vi "createCommandParameters.vi"(8 "error in (no error)":errorcluster, 9 "value":variant, 10 "command":T1, 11 "CoolerSerialCommand in":refnum<class "CoolerSerialCommand.lvclass">) -> (0 "error out":errorcluster, 1 "commandName":string, 2 "commandId":string, 3 "CoolerSerialCommand out":refnum<class "CoolerSerialCommand.lvclass">, 5 "cmdData":string)   [LabVIEW 2016, in "CoolerSerialCommand.lvclass"]
uses:
  CoolerSerialCommand.lvclass
  typedefs/CoolerCommands.ctl
  typedefs/dataType.ctl
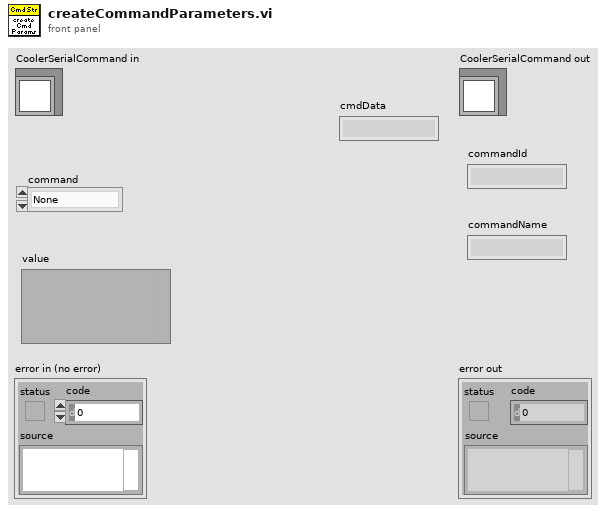
[diagram p1: front panel]
types:
  T1 = typedef "CoolerCommands.ctl" = enum16{"None", "SetExternSensorStatus", "SetChillerStatus", "SetControlSensor", "SetControlTemperature", "SetHighSupplyTempWarning", "SetLowSupplyTemperatureWarning", "SetHighAmbientTemperatureWarning", "SetLowAmbienTemperatureWarning", "SetLowProcessFlowWarning", "SetHighSupplyTemperatureAlarm", "SetLowSupplyTemperatureAlarm", "SetHighAmbientTemperatureAlarm", "SetLowAmbientTemperatureAlarm", "SetLowProcessFlowAlarm"}
  T2 = typedef "dataType.ctl" = enum16{"Temperature", "Flow", "ControlSensor", "ExternalSensorStatus", "ChillerStatus"}
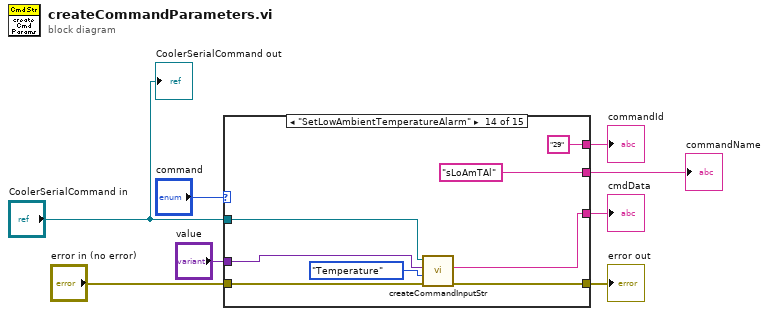
[diagram p0: block diagram]
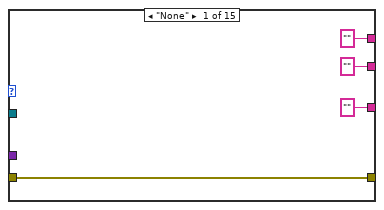
[diagram p2: hidden frame]
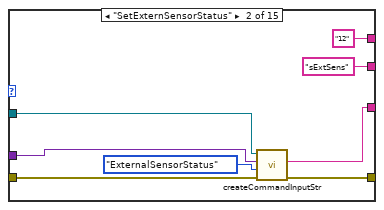
[diagram p3: hidden frame]
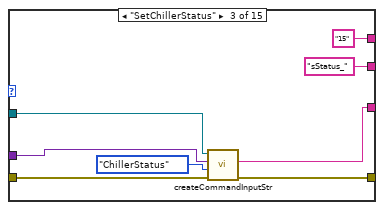
[diagram p4: hidden frame]
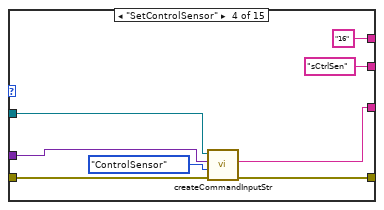
[diagram p5: hidden frame]
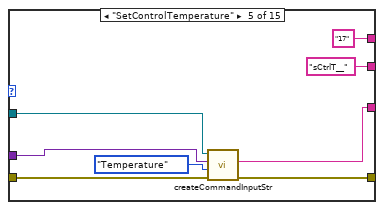
[diagram p6: hidden frame]
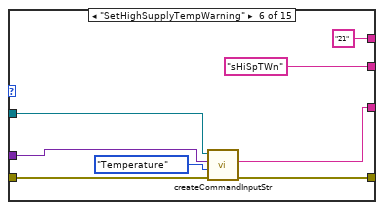
[diagram p7: hidden frame]
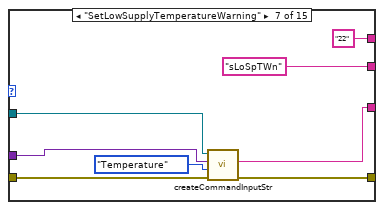
[diagram p8: hidden frame]
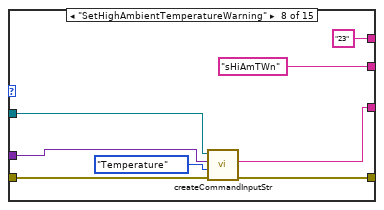
[diagram p9: hidden frame]
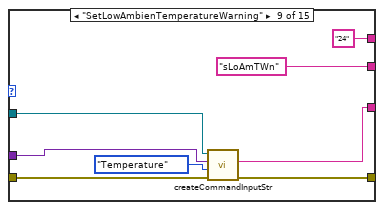
[diagram p10: hidden frame]
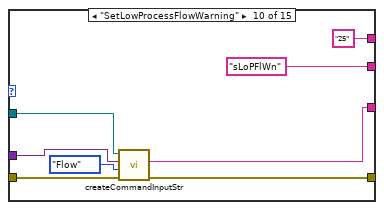
[diagram p11: hidden frame]
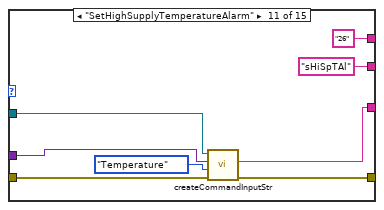
[diagram p12: hidden frame]
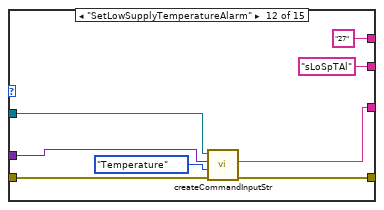
[diagram p13: hidden frame]
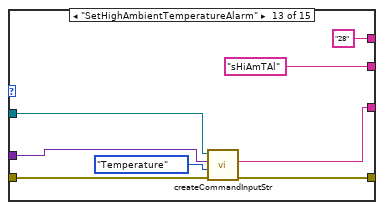
[diagram p14: hidden frame]
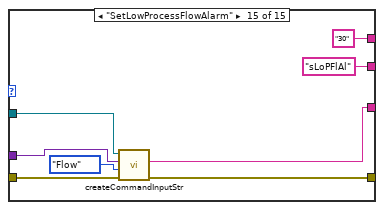
[diagram p15: hidden frame]
diagram:
  n1 = case shown="\"SetLowAmbientTemperatureAlarm\"" "command" {
    tunnel: ["" ("commandId") "12" ("commandId") "15" ("commandId") "16" ("commandId") "17" ("commandId") "21" ("commandId") "22" ("commandId") "23" ("commandId") "24" ("commandId") "25" ("commandId") "26" ("commandId") "27" ("commandId") "28" ("commandId") "29" ("commandId") "30" ("commandId")] -> w7
    tunnel: ["" ("commandId") "sExtSens" ("commandId") "sStatus_" ("commandId") "sCtrlSen" ("commandId") "sCtrlT__" ("commandId") "sHiSpTWn" ("commandId") "sLoSpTWn" ("commandId") "sHiAmTWn" ("commandId") "sLoAmTWn" ("commandId") "sLoPFlWn" ("commandId") "sHiSpTAl" ("commandId") "sLoSpTAl" ("commandId") "sHiAmTAl" ("commandId") "sLoAmTAl" ("commandId") "sLoPFlAl" ("commandId")] -> w6
    tunnel: "value" -> [_ w18 w21 w33 w38 w46 w54 w62 w70 w78 w85 w97 w105 w113 w120]
    tunnel: "error in (no error)" -> [w9 w17 w25 w31 w37 w45 w53 w61 w69 w77 w89 w96 w104 w112 w119]
    tunnel: [w9 w14 w24 w29 w41 w49 w56 w64 w72 w80 w88 w95 w103 w111 w118] -> w3
    tunnel: ["" ("cmdDataStr") w13 w22 w30 w42 w50 w57 w66 w73 w81 w87 w94 w102 w110 w117] -> w2
    tunnel: "CoolerSerialCommand in" -> [_ w15 w26 w34 w40 w48 w58 w65 w74 w82 w86 w93 w101 w109 w121]
    frame "None" {
    }
    frame "SetExternSensorStatus" {
      n2 = call "createCommandInputStr.vi"("error in (no error)"=w17, "dataType"=dataType."ExternalSensorStatus", "data"=w18, "CoolerSerialCommand in"=w15) -> ("error out"=w14:errorcluster, "cmdDataStr"=w13:string)  [unwired: 5 in, 1 out]
    }
    frame "SetChillerStatus" {
      n3 = call "createCommandInputStr.vi"("error in (no error)"=w25, "dataType"=dataType."ChillerStatus", "data"=w21, "CoolerSerialCommand in"=w26) -> ("error out"=w24:errorcluster, "cmdDataStr"=w22:string)  [unwired: 5 in, 1 out]
    }
    frame "SetControlSensor" {
      n4 = call "createCommandInputStr.vi"("error in (no error)"=w31, "dataType"=dataType."ControlSensor", "data"=w33, "CoolerSerialCommand in"=w34) -> ("error out"=w29:errorcluster, "cmdDataStr"=w30:string)  [unwired: 5 in, 1 out]
    }
    frame "SetControlTemperature" {
      n5 = call "createCommandInputStr.vi"("error in (no error)"=w37, "dataType"=dataType."Temperature", "data"=w38, "CoolerSerialCommand in"=w40) -> ("error out"=w41:errorcluster, "cmdDataStr"=w42:string)  [unwired: 5 in, 1 out]
    }
    frame "SetHighSupplyTempWarning" {
      n6 = call "createCommandInputStr.vi"("error in (no error)"=w45, "dataType"=dataType."Temperature", "data"=w46, "CoolerSerialCommand in"=w48) -> ("error out"=w49:errorcluster, "cmdDataStr"=w50:string)  [unwired: 5 in, 1 out]
    }
    frame "SetLowSupplyTemperatureWarning" {
      n7 = call "createCommandInputStr.vi"("error in (no error)"=w53, "dataType"=dataType."Temperature", "data"=w54, "CoolerSerialCommand in"=w58) -> ("error out"=w56:errorcluster, "cmdDataStr"=w57:string)  [unwired: 5 in, 1 out]
    }
    frame "SetHighAmbientTemperatureWarning" {
      n8 = call "createCommandInputStr.vi"("error in (no error)"=w61, "dataType"=dataType."Temperature", "data"=w62, "CoolerSerialCommand in"=w65) -> ("error out"=w64:errorcluster, "cmdDataStr"=w66:string)  [unwired: 5 in, 1 out]
    }
    frame "SetLowAmbienTemperatureWarning" {
      n9 = call "createCommandInputStr.vi"("error in (no error)"=w69, "dataType"=dataType."Temperature", "data"=w70, "CoolerSerialCommand in"=w74) -> ("error out"=w72:errorcluster, "cmdDataStr"=w73:string)  [unwired: 5 in, 1 out]
    }
    frame "SetLowProcessFlowWarning" {
      n10 = call "createCommandInputStr.vi"("error in (no error)"=w77, "dataType"=dataType."Flow", "data"=w78, "CoolerSerialCommand in"=w82) -> ("error out"=w80:errorcluster, "cmdDataStr"=w81:string)  [unwired: 5 in, 1 out]
    }
    frame "SetHighSupplyTemperatureAlarm" {
      n11 = call "createCommandInputStr.vi"("error in (no error)"=w89, "dataType"=dataType."Temperature", "data"=w85, "CoolerSerialCommand in"=w86) -> ("error out"=w88:errorcluster, "cmdDataStr"=w87:string)  [unwired: 5 in, 1 out]
    }
    frame "SetLowSupplyTemperatureAlarm" {
      n12 = call "createCommandInputStr.vi"("error in (no error)"=w96, "dataType"=dataType."Temperature", "data"=w97, "CoolerSerialCommand in"=w93) -> ("error out"=w95:errorcluster, "cmdDataStr"=w94:string)  [unwired: 5 in, 1 out]
    }
    frame "SetHighAmbientTemperatureAlarm" {
      n13 = call "createCommandInputStr.vi"("error in (no error)"=w104, "dataType"=dataType."Temperature", "data"=w105, "CoolerSerialCommand in"=w101) -> ("error out"=w103:errorcluster, "cmdDataStr"=w102:string)  [unwired: 5 in, 1 out]
    }
    frame "SetLowAmbientTemperatureAlarm" {
      n14 = call "createCommandInputStr.vi"("error in (no error)"=w112, "dataType"=dataType."Temperature", "data"=w113, "CoolerSerialCommand in"=w109) -> ("error out"=w111:errorcluster, "cmdDataStr"=w110:string)  [unwired: 5 in, 1 out]
    }
    frame "SetLowProcessFlowAlarm" {
      n15 = call "createCommandInputStr.vi"("error in (no error)"=w119, "dataType"=dataType."Flow", "data"=w120, "CoolerSerialCommand in"=w121) -> ("error out"=w118:errorcluster, "cmdDataStr"=w117:string)  [unwired: 5 in, 1 out]
    }
  }
  "error out" <- w3
  "commandId" <- w7
  "commandName" <- w6
  "cmdData" <- w2
  "CoolerSerialCommand out" <- "CoolerSerialCommand in"
